vi "Add Documentation to Constructor VI.vi"   [LabVIEW 2015]
doc: "<b> </b> <b> </b>\n©2016 Q Software Innovations, LLC (QSI)\nwritten by Quentin Alldredge\nproduced in LabVIEW 2015"
uses:
  Project Manipulation Scripts/Project Manipulation Scripts.lvlib
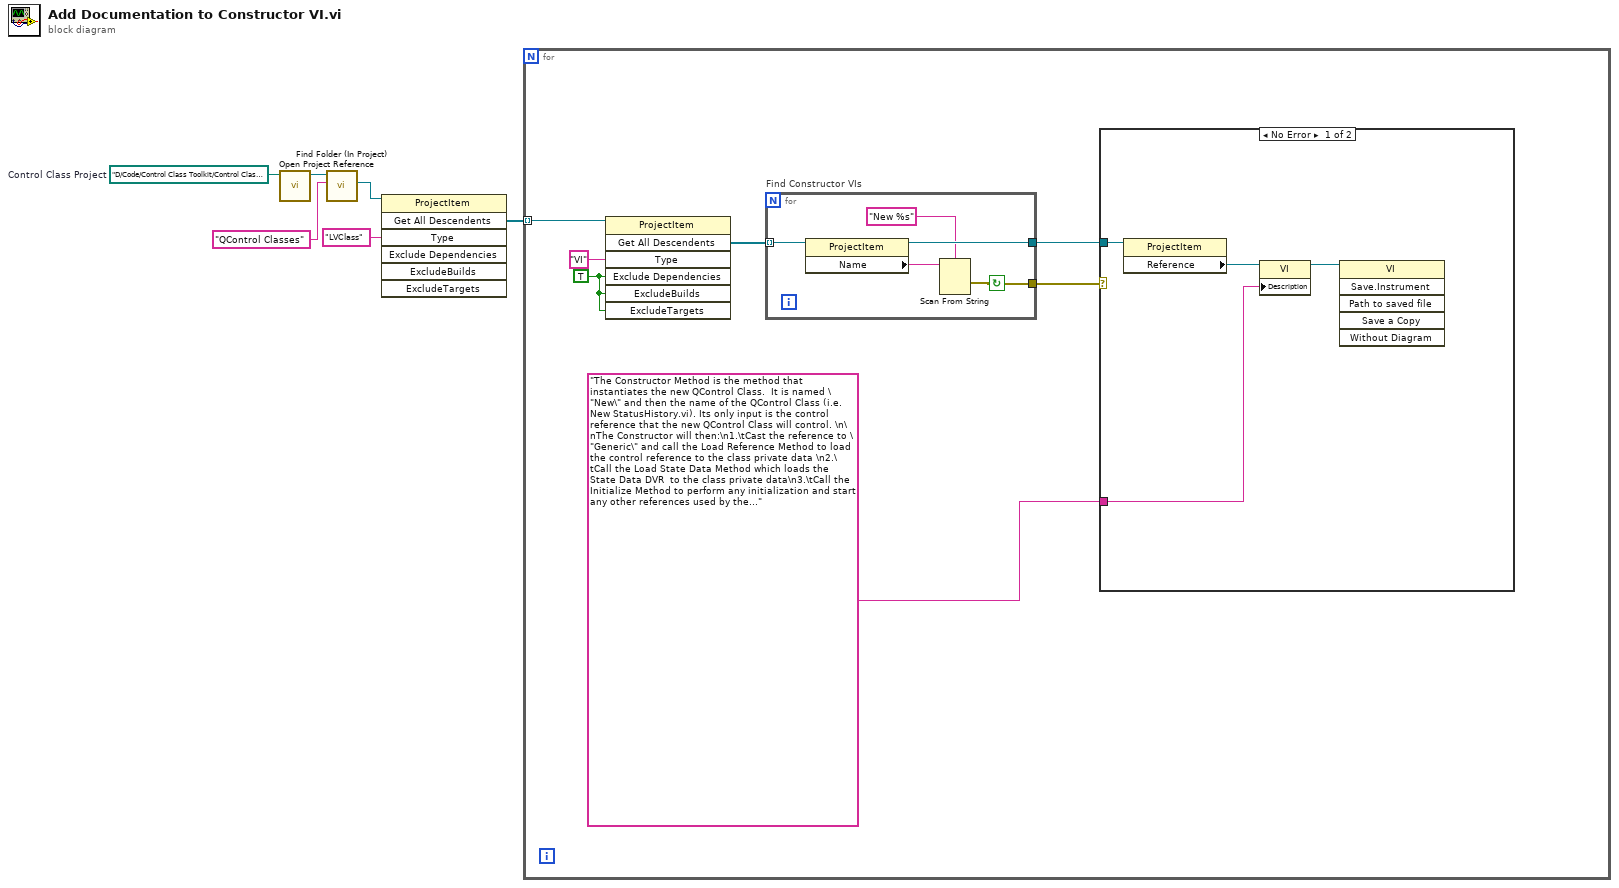
[diagram p0: block diagram]
diagram:
  w6 = path "D:/Code/Control Class Toolkit/Control Class Toolkit.lvproj"  # Control Class Project
  n1 = call "Open Project Reference.vi"("Project Path"=w6) -> ("Project out"=w5:refnum<vi>)  [unwired: 10 in]
  n2 = call "Find Folder (In Project).vi"("Folder Name"="QControl Classes", "Project in"=w5) -> ("Folder Refnum"=w3:refnum<vi>)  [unwired: 7 in, 2 out]
  n3 = invoke class="ProjectItem" method="Get All Descendents"(reference=w3, "Type"="LVClass") -> ("All Descendents"=w1:refnum<vi>[])  [unwired: 5 in, 6 out]
  n4 = for {
    tunnel: w1 -> [w8] mode=indexing
    w11 = TRUE ("ExcludeDependencies")
    n5 = invoke class="ProjectItem" method="Get All Descendents"(reference=w8, "Type"="VI", "Exclude Dependencies"=w11, "ExcludeBuilds"=w11, "ExcludeTargets"=w11) -> ("All Descendents"=w13:refnum<vi>[])  [unwired: 2 in, 6 out]
    n6 = for "Find Constructor VIs" {
      tunnel: w13 -> [w18] mode=indexing
      tunnel: [w17] -> w9
      tunnel: [w14] -> w10
      stop <- w14 continue-if-true
      n7 = property class="ProjectItem"(reference=w18) -> (reference out=w17:refnum<vi>, "Name"=w16:string)  [unwired: 1 in, 1 out]
      n8 = Scan From String(format string="New %s", input string=w16) -> (error out=w14:errorcluster)  [unwired: 4 in, 2 out]
    }
    n9 = case shown="No Error" w10 {
      tunnel: w9 -> [w22 _]
      tunnel: "The Constructor Method is the method that instantiates the new QControl Class.  It is named \"New\" and then the name of the QControl Class (i.e. New StatusHistory.vi). Its only input is the control reference that the new QControl Class will control. \n\nThe Constructor will then:\n1.\tCast the reference to \"Generic\" and call the Load Reference Method to load the control reference to the class private data \n2.\tCall the Load State Data Method which loads the State Data DVR  to the class private data\n3.\tCall the Initialize Method to perform any initialization and start any other references used by the QControl Class and launch the Event Handler\n\nThe output of the Constructor Method is the QControl Class Wire.  This wire should be handled and passed just like the reference of a basic control/indicator.  <b>Any manipulation of the control after the Constructor Method should use Properties or Methods on this wire or handle UI Logic in the Event Handler.</b>\n \n<b> </b> <b> </b>\n©2016 Q Software Innovations, LLC  (QSI)\nwritten by Quentin Alldredge\nproduced in LabVIEW 2015 " ("VI Description") -> [w20 _]
      frame No Error {
        n10 = property class="ProjectItem"(reference=w22) -> ("Reference"=w21:refnum<vi>)  [unwired: 1 in, 2 out]
        n11 = property class="VI"(reference=w21, "Description"=w20) -> (reference out=w19:refnum<vi>)  [unwired: 1 in, 1 out]
        n12 = invoke class="VI" method="Save.Instrument"(reference=w19) -> ()  [unwired: 5 in, 6 out]
      }
      frame Error {
      }
    }
  }
